vi "interpolate_hadamard_to_frames.vi"(1 "Hadamard":bool[][](array[boolean])) -> (0 "Fames":u8[][][](array[numeric]))   [LabVIEW 2020]
uses:
  <vilib>/Analysis/baseanly.llb/Mean (DBL).vi
  <vilib>/Analysis/NI_AALBase.lvlib
panel:
  out "Time/iteration":dbl
  out "Resamples":i32[](array[numeric])
  out "Letterbox 1":dbl format="%0.2f"
  out "Scale":dbl format="%0.2f"
  out "Total":dbl format="%0.2f"
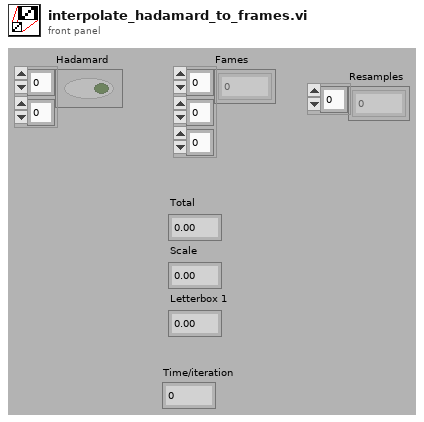
[diagram p1: front panel]
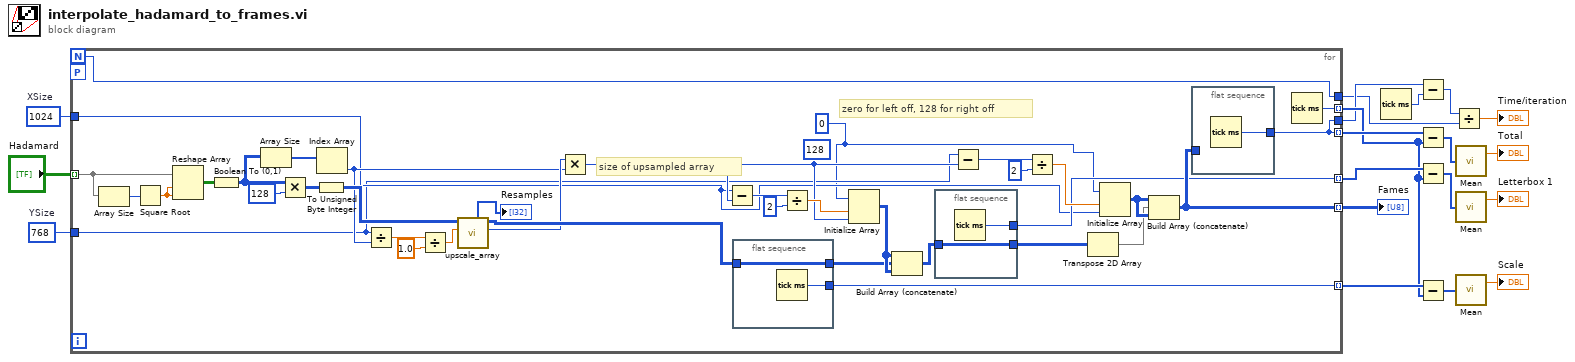
[diagram p0: block diagram]
diagram:
  w18 = 1024  # XSize
  w17 = 768  # YSize
  n1 = for {
    N -> [w25]
    tunnel: "Hadamard" -> [w56] mode=indexing
    tunnel: w18 -> [w27]
    tunnel: w17 -> [w26]
    tunnel: [w54] -> w16 mode=indexing
    tunnel: [w34] -> w7 mode=indexing
    tunnel: [w32] -> w12 mode=indexing
    tunnel: [w31] -> w10 mode=indexing
    tunnel: [w24] -> w8 mode=indexing
    tunnel: [w25] -> w2
    tunnel: [w24] -> w5
    workers-P: _ -> [_]
    w20 = u8 0 ("element")
    (unwired) u8 128 ("element")
    # "zero for left off, 128 for right off"
    # "size of upsampled array"
    n2 = Array Size(array=w56) -> (size(s)=w57:i32)
    n3 = Square Root(x=w57) -> (sqrt(x)=w55:dbl)
    n4 = Reshape Array(w56, w55, w55) -> (w37:bool[][])
    n5 = Boolean To (0,1)(Boolean=w37) -> (0, 1=w50:i16[][])
    n6 = Array Size(array=w50) -> (size(s)=w51:i32[])
    n7 = Multiply(x=w50, y=u8 128) -> (x*y=w52:i16[][])
    n8 = To Unsigned Byte Integer(number=w52) -> (unsigned 8bit integer=w39:u8[][])
    n9 = Index Array(array=w51) -> (element=w29:i32)  [unwired: 1 in]
    n10 = Divide(x=w26, y=w29) -> (x/y=w23:dbl)
    n11 = Divide(x=w23, y=1.0) -> (x/y=w21:dbl)
    n12 = call "upscale_array.vi"("Upsample Factor"=w21, "Small Array"=w39) -> ("Actual Upsample Factor"=w30:i32, "Big Array"=w36:u8[][], "Resamples"=→"Resamples":i32[])  [unwired: 7 in]
    n13 = Multiply(x=w30, y=w29) -> (x*y=w28:i32)
    n14 = Subtract(x=w27, y=w28) -> (x-y=w49:i32)
    n15 = flat-sequence {
      tunnel: [w62] -> w32
      tunnel: w36 -> [w61]
      tunnel: [w61] -> w35
      frame #0 {
        n16 = Tick Count (ms)() -> (millisecond timer value=w62:u32)
      }
    }
    n17 = Divide(x=w49, y=2) -> (x/y=w47:dbl)
    n18 = Initialize Array(w20, w47, w28) -> (w46:u8[][])
    n19 = Build Array (concatenate)(w46, w35, w46) -> (w41:u8[][])
    n20 = flat-sequence {
      tunnel: [w60] -> w31
      tunnel: w41 -> [w59]
      tunnel: [w59] -> w40
      frame #0 {
        n21 = Tick Count (ms)() -> (millisecond timer value=w60:u32)
      }
    }
    n22 = Subtract(x=w26, y=w28) -> (x-y=w42:i32)
    n23 = Divide(x=w42, y=2) -> (x/y=w44:dbl)
    n24 = Transpose 2D Array(2D array=w40) -> (transposed array=w33:u8[][])
    n25 = Initialize Array(w20, w44, w27) -> (w45:u8[][])
    n26 = Build Array (concatenate)(w45, w33, w45) -> (w54:u8[][])
    n27 = flat-sequence {
      tunnel: [w58] -> w24
      tunnel: w54 -> [_]
      frame #0 {
        n28 = Tick Count (ms)() -> (millisecond timer value=w58:u32)
      }
    }
    n29 = Tick Count (ms)() -> (millisecond timer value=w34:u32)
  }
  "Fames" <- w16
  n30 = Tick Count (ms)() -> (millisecond timer value=w4:u32)
  n31 = Subtract(x=w5, y=w4) -> (x-y=w3:u32)
  n32 = Subtract(x=w8, y=w7) -> (x-y=w6:u32[])
  n33 = Subtract(x=w10, y=w7) -> (x-y=w9:u32[])
  n34 = Subtract(x=w12, y=w7) -> (x-y=w11:u32[])
  n35 = Divide(x=w3, y=w2) -> (x/y=→"Time/iteration":dbl)
  n36 = call-poly <vilib>:"Mean.vi"("X"=w6) -> ("mean"=→"Total":dbl)  [unwired: 1 out]
  n37 = call-poly <vilib>:"Mean.vi"("X"=w9) -> ("mean"=→"Letterbox 1":dbl)  [unwired: 1 out]
  n38 = call-poly <vilib>:"Mean.vi"("X"=w11) -> ("mean"=→"Scale":dbl)  [unwired: 1 out]
